vi "test_toml_writer.vi"(8 "error in (no error)":errorcluster, 11 "toml_string in":string="\n[project.stuff]\nname = \"jim's project\"\nversion = \"0.1.0\"\n\n[nipm]\nversion = \"1.2.3\"\n\n[nipm.dependencies]\nmy_package2 = { version = \"1.2.3\" }\nni-daqmx = { version = \"1.0\" , url = \"ni.com\" , \"\" = \"\" }\n\n[vipm]\n\n[vipm.dependencies]\noglib_array = { version = \"6.5.4\", url = \"https://jki.net\"}\noglib_string = \"3.1.4\"\n\n\n\n") -> ()   [LabVIEW 2020]
uses:
  toml/toml.lvclass
panel:
  out "original_value":string="6.6.6"
  out "value":string="6.6.6"
  out "toml_string out":string
  out "error out":errorcluster
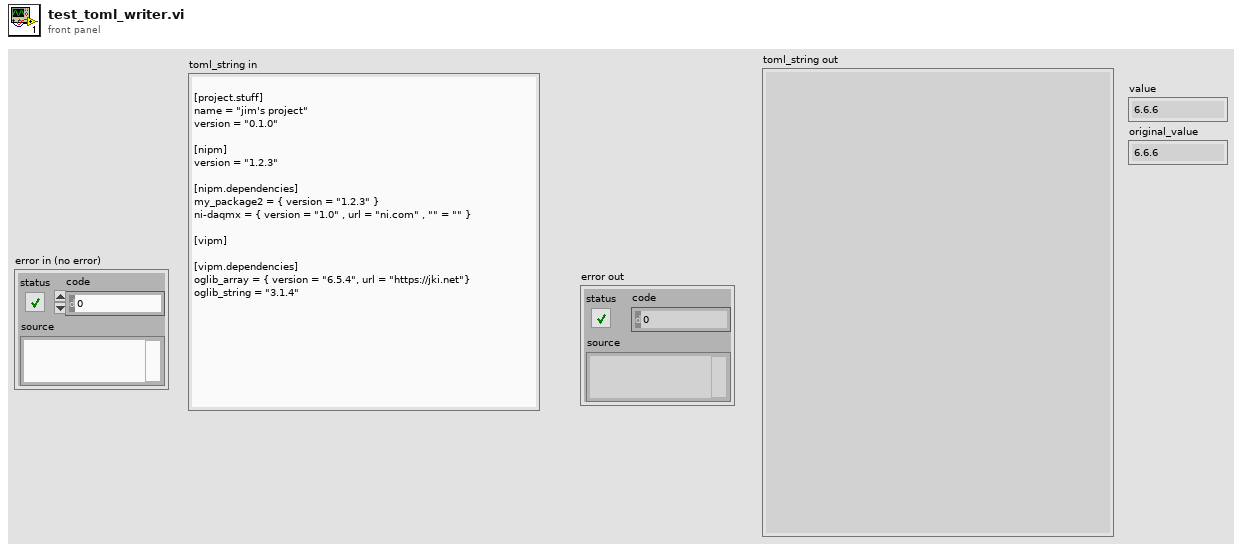
[diagram p1: front panel]
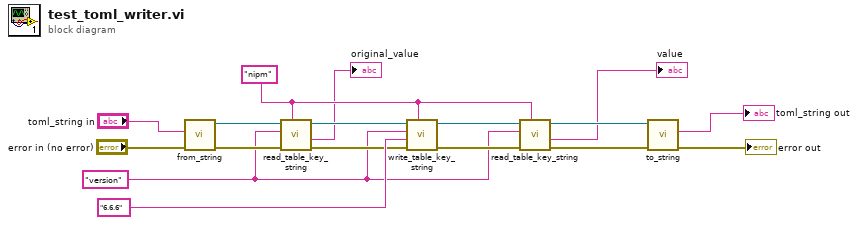
[diagram p0: block diagram]
diagram:
  w2 = "version" ("table_name")
  w3 = "nipm" ("table_name")
  n1 = call "from_string.vi"("error in (no error)"="error in (no error)", "toml"="toml_string in") -> ("error out"=w7:errorcluster, "toml out"=w6:refnum<class "toml.lvclass">)  [unwired: 8 in]
  n2 = call "read_table_key_string.vi"("table"=w3, "error in (no error)"=w7, "key"=w2, "toml in"=w6) -> ("error out"=w4:errorcluster, "value"=→"original_value":string, "toml out"=w5:refnum<class "toml.lvclass">)  [unwired: 5 in]
  n3 = call "write_table_key_string.vi"("table"=w3, "error in (no error)"=w4, "value"="6.6.6" ("string"), "key"=w2, "toml in"=w5) -> ("error out"=w12:errorcluster, "toml out"=w10:refnum<class "toml.lvclass">)  [unwired: 5 in]
  n4 = call "read_table_key_string.vi"("table"=w3, "error in (no error)"=w12, "key"=w2, "toml in"=w10) -> ("error out"=w11:errorcluster, "value"=→"value":string, "toml out"=w9:refnum<class "toml.lvclass">)  [unwired: 5 in]
  n5 = call "to_string.vi"("error in (no error)"=w11, "toml in"=w9) -> ("error out"=→"error out":errorcluster, "toml_string"=→"toml_string out":string)  [unwired: 8 in]
